vi "Autosave.vi"(8 "error in (no error)":errorcluster, 9 "Base Name":string, 10 "Save Cluster":T1 {"Select Layout" items=["Default"]}, 11 "Autosave Path":path=path "") -> (0 "error out (passthrough)":errorcluster, 2 "Autosave Success":bool)   [LabVIEW 2013]
uses:
  TypeDefs/SaveCluster.ctl
  VariableManagerCodes/VariableManager/VariableManager.lvclass
  DeviceVIs/Device/Device.lvclass
  <vilib>/Utility/miscctls.llb/LVStringsAndValuesArrayTypeDef_I32.ctl
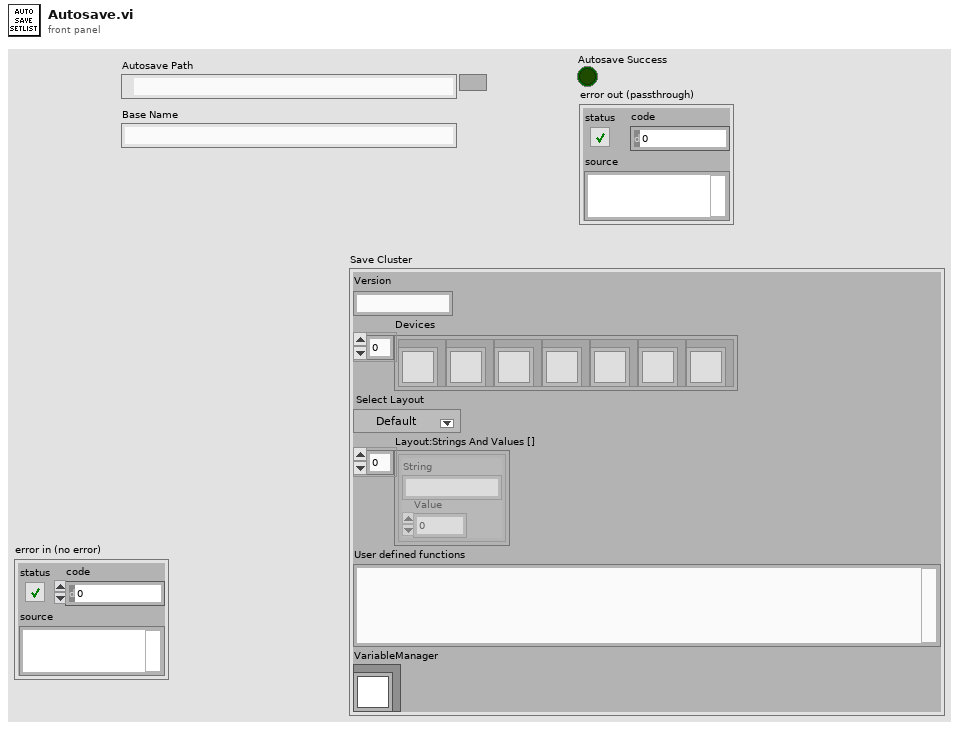
[diagram p1: front panel]
types:
  T1 = typedef "SaveCluster.ctl" = cluster{"Version":string, "Devices":refnum<class "Device.lvclass">[], "Select Layout":i32, "Layout:Strings And Values []":T2, "User defined functions":string, "VariableManager":refnum<class "VariableManager.lvclass">}
  T2 = typedef "LVStringsAndValuesArrayTypeDef_I32.ctl" = cluster{"String":string, "Value":i32}[]
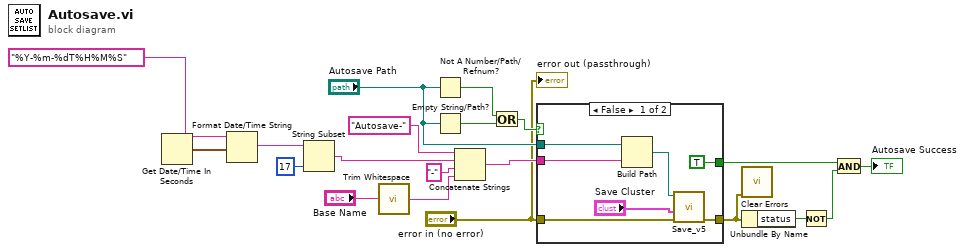
[diagram p0: block diagram]
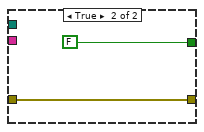
[diagram p2: hidden frame]
diagram:
  n1 = Get Date/Time In Seconds() -> (seconds since 1Jan1904=w5:timestamp)
  n2 = Format Date/Time String(time format string (%c)="%Y-%m-%dT%H%M%S", seconds (now)=w5) -> (date/time string=w3:string)  [unwired: 1 in]
  n3 = String Subset(string=w3, length (rest)=17 ("length (rest)")) -> (substring=w1:string)  [unwired: 1 in]
  n4 = call <vilib>:"Trim Whitespace.vi"("string"="Base Name") -> ("trimmed string"=w6:string)  [unwired: 1 in]
  n5 = Not A Number/Path/Refnum?(number/path/refnum="Autosave Path") -> (NaN/Path/Refnum?=w18:bool)
  n6 = Empty String/Path?(string/path="Autosave Path") -> (empty?=w17:bool)
  n7 = Concatenate Strings("Autosave-" ("string"), w1, "-" ("string"), w6) -> (w15:string)
  n8 = Or(x=w18, y=w17) -> (x .or. y?=w16:bool)
  n9 = case shown="False" w16 {
    tunnel: "error in (no error)" -> [w27 w29]
    tunnel: [w23 w29] -> w13
    tunnel: "Autosave Path" -> [w24 _]
    tunnel: w15 -> [w21 _]
    tunnel: [TRUE FALSE] -> w10
    frame False {
      n10 = Build Path(base path=w24, name or relative path=w21) -> (appended path=w26:path)
      n11 = call "Save_v5.vi"("error in"=w27, "Save Cluster"="Save Cluster", "Path (open dialog)"=w26) -> ("error out"=w23:errorcluster)  [unwired: 5 in, 3 out]
    }
    frame True {
    }
  }
  n12 = call <vilib>:"Clear Errors.vi"("error in (no error)"=w13) -> ()  [unwired: 6 in, 1 out]
  n13 = Unbundle By Name(w13) -> ("status"=w12:bool)
  n14 = Not(x=w12) -> (.not. x?=w11:bool)
  n15 = And(x=w10, y=w11) -> (x .and. y?=→"Autosave Success":bool)
  "error out (passthrough)" <- "error in (no error)"
